vi "全局F结果.vi"() -> ()   [LabVIEW 2018]
panel:
  out "3#拨钮下上力检":cluster{"判断完成":bool, "不合格?":bool}
  out "3#拨钮上下力检":cluster{"判断完成":bool, "不合格?":bool}
  out "3#拨钮右左力检":cluster{"判断完成":bool, "不合格?":bool}
  out "3#拨钮左右力检":cluster{"判断完成":bool, "不合格?":bool}
  out "3#轮盘开关力检":cluster{"判断完成":bool, "不合格?":bool}
  out "3#轮盘关开力检":cluster{"判断完成":bool, "不合格?":bool}
  out "2#拨钮下上力检":cluster{"判断完成":bool, "不合格?":bool}
  out "2#拨钮上下力检":cluster{"判断完成":bool, "不合格?":bool}
  out "2#拨钮右左力检":cluster{"判断完成":bool, "不合格?":bool}
  out "2#拨钮左右力检":cluster{"判断完成":bool, "不合格?":bool}
  out "2#轮盘开关力检":cluster{"判断完成":bool, "不合格?":bool}
  out "2#轮盘关开力检":cluster{"判断完成":bool, "不合格?":bool}
  out "1#拨钮下上力检":cluster{"判断完成":bool, "不合格?":bool}
  out "1#拨钮上下力检":cluster{"判断完成":bool, "不合格?":bool}
  out "1#拨钮右左力检":cluster{"判断完成":bool, "不合格?":bool}
  out "1#拨钮左右力检":cluster{"判断完成":bool, "不合格?":bool}
  out "1#轮盘开关力检":cluster{"判断完成":bool, "不合格?":bool}
  out "1#轮盘关开力检":cluster{"判断完成":bool, "不合格?":bool}
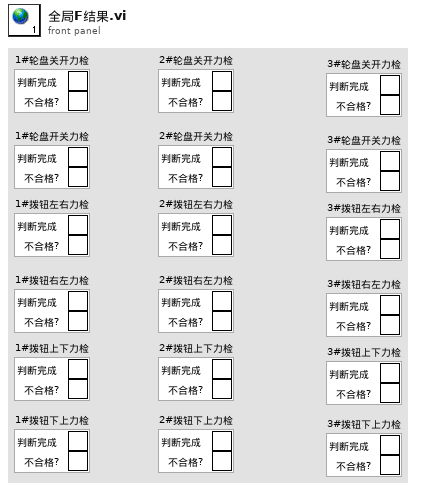
[diagram p1: front panel]
diagram:
